vi "Open.vi"(8 "error in":errorcluster, 9 "parameters":variant, 10 "file path":path, 11 "repository in":refnum<class "modification container.lvclass">) -> (0 "error out":errorcluster, 2 "invalid?":bool, 3 "repository out":refnum<class "modification container.lvclass">)   [LabVIEW 2013, in "modification container.lvclass"]
doc: "Loads the saved information of the repo. It could load multiple files at the same time. An option to add file versioning could be included in the files, and the code to manage changes would be in this VI."
uses:
  modification container.lvclass
  FileCluster.ctl
  VI modification.lvclass
  modification container.lvclass/modification container.ctl
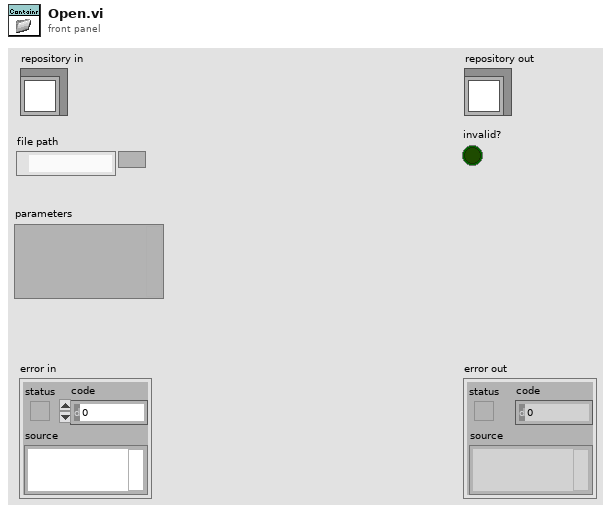
[diagram p1: front panel]
types:
  T1 = typedef "modification container.lvclass/FileCluster.ctl" = cluster{"Version":string, "Data":variant}
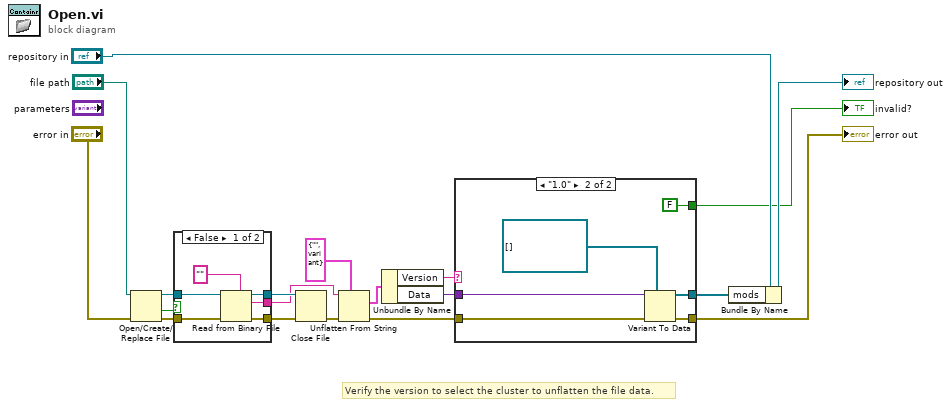
[diagram p0: block diagram]
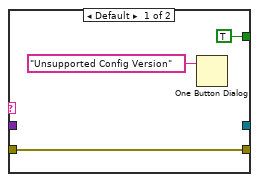
[diagram p2: hidden frame]
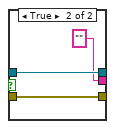
[diagram p3: hidden frame]
diagram:
  # "Verify the version to select the cluster to unflatten the file data."
  n1 = Open/Create/Replace File(file path (use dialog)="file path", error in="error in") -> (refnum out=w18:refnum<file>, cancelled=w19:bool, error out=w15:errorcluster)  [unwired: 4 in]
  n2 = case shown="False" w19 {
    tunnel: w18 -> [w25 w28]
    tunnel: [w24 w28] -> w17
    tunnel: [w23 w27] -> w16
    tunnel: w15 -> [w22 w27]
    tunnel: [w21 ""] -> w13
    frame False {
      n3 = Read from Binary File(5:"" ("data type"), 8:w22, 11:w25) -> (0:w23:errorcluster, 2:w21:string, 3:w24:refnum<file>)  [unwired: 3 in, 1 out]
    }
    frame True {
    }
  }
  n4 = Close File(refnum=w17, error in=w16) -> (error out=w9:errorcluster)  [unwired: 1 out]
  n5 = Unflatten From String(type=T1 {"Version"="", "Data"=variant}, binary string=w13, error in (no error)=w9) -> (value=w7:T1, error out=w10:errorcluster)  [unwired: 2 in, 1 out]
  n6 = Unbundle By Name(w7) -> ("Version"=w12:string, "Data"=w11:variant)
  n7 = case shown="\"1.0\"" w12 {
    tunnel: [_ w37] -> w8
    tunnel: [w31 w36] -> w3
    tunnel: w10 -> [w31 w33]
    tunnel: w11 -> [_ w34]
    tunnel: [TRUE FALSE] -> w1
    frame Default {
      n8 = One Button Dialog(message="Unsupported Config Version") -> ()  [unwired: 1 in, 1 out]
    }
    frame "1.0" {
      n9 = Variant To Data(error in=w33, type=refnum<class "VI modification.lvclass">[] [] ("mods"), Variant=w34) -> (data=w37:refnum<class "VI modification.lvclass">[], error out=w36:errorcluster)
    }
  }
  "error out" <- w3
  "invalid?" <- w1
  n10 = Bundle By Name(cluster="repository in", "mods"=w8) -> (→"repository out":refnum<class "modification container.lvclass">)
